vi "ma_SML Decimation Filter (complex input).vi"(2 "reset?":bool, 3 "truncate transition?":bool=TRUE, 4 "decimation setting":T1={"M"=1, "stop band attenuation"=enum."84 dB", "alias protect in transition band"=TRUE, "oversampling ratio"=1.0} {"oversampling ratio" format="%.2f"; "M" min=0}, 5 "x":cdb[](array[numeric]) format="%.2f") -> (0 "initial cutoff length":i32=1 min=0, 1 "y":cdb[](array[numeric]) format="%.2f")   [LabVIEW 2020, in "NI_MAPro.lvlib"]
uses:
  NI_MAPro.lvlib
  NI_AALPro.lvlib
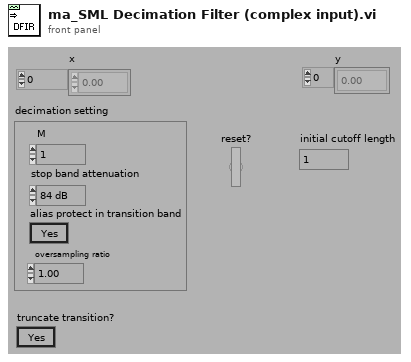
[diagram p1: front panel]
types:
  T1 = cluster{"M":i32, "stop band attenuation":enum16{"84 dB", "96 dB", "120 dB"}, "alias protect in transition band":bool, "oversampling ratio":dbl}
  T2 = cluster{"M":bool, "stop band attenuation":bool, "alias protect in transition band":bool, "oversampling ratio":bool}
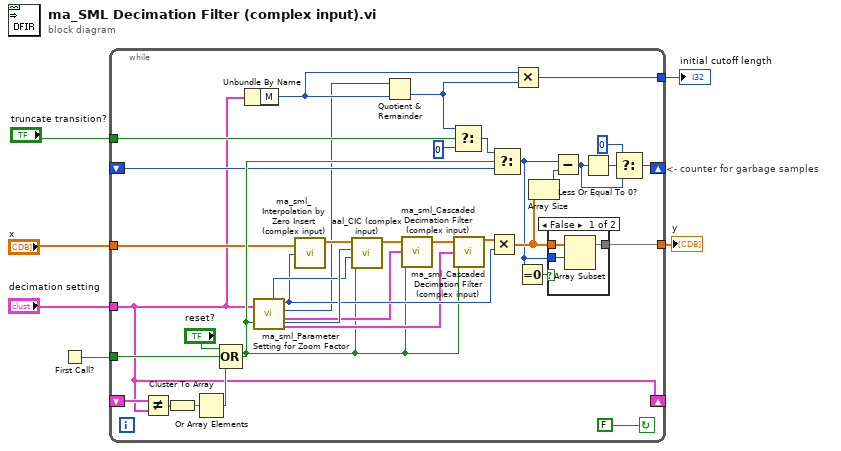
[diagram p0: block diagram]
diagram:
  # "<- counter for garbage samples"
  n1 = First Call?() -> (First Call?: T/F=w3:bool)
  n2 = while {
    tunnel: [w10] -> w1
    tunnel: "truncate transition?" -> [w12]
    tunnel: w3 -> [w13]
    tunnel: "x" -> [w18]
    tunnel: "decimation setting" -> [w11]
    shift-left: _ -> [w27]
    shift-right: [w23] -> _
    tunnel: [w30] -> w6
    shift-left: _ -> [w34]
    shift-right: [w11] -> _
    stop <- FALSE continue-if-true
    n3 = Not Equal?(x=w34, y=w11) -> (x != y?=w33:T2)
    n4 = Cluster To Array(cluster=w33) -> (array=w32:bool[])
    n5 = Or Array Elements(Boolean array=w32) -> (logical OR=w14:bool)
    n6 = Compound Arithmetic op=OR("reset?", w13, w14) -> (w28:bool)
    n7 = Unbundle By Name(w11) -> ("M"=w8:i32)
    n8 = call "ma_sml_Parameter Setting for Zoom Factor.vi"("zoom settings"=w11, "Reset"=w28) -> ("CIC Stages"=w40:i32, "comb filter order"=w41:i32, "interpolation"=w39:i32, "filter length"=w7:i32, "CFIR par"=w29:cluster{"h":dbl[], "M":i32, "N":i32}, "LFIR par"=w35:cluster{"h":dbl[], "M":i32, "N":i32})
    n9 = call "ma_sml_Interpolation by Zero Insert (complex input).vi"("L"=w39, "x"=w18) -> ("y"=w42:cdb[])
    n10 = call "aal_CIC (complex input).vi"("Reset"=w28, "Stages"=w40, "N"=w41, "x"=w42) -> ("y"=w36:cdb[])
    n11 = Quotient & Remainder(x=w7, y=w8) -> (floor(x/y)=w9:i32)  [unwired: 1 out]
    n12 = call "ma_sml_Cascaded Decimation Filter (complex input).vi"("reset?"=w28, "filter specification"=w29, "x"=w36) -> ("y"=w38:cdb[])
    n13 = Select(t=w9, s=w12, f=0) -> (s? t:f=w16:i32)
    n14 = call "ma_sml_Cascaded Decimation Filter (complex input).vi"("reset?"=w28, "filter specification"=w35, "x"=w38) -> ("y"=w37:cdb[])
    n15 = Multiply(x=w37, y=w39) -> (x*y=w26:cdb[])
    n16 = Select(t=w16, s=w28, f=w27) -> (s? t:f=w20:i32)
    n17 = Multiply(x=w8, y=w9) -> (x*y=w10:i32)
    n18 = Equal To 0?(x=w20) -> (x = 0?=w19:bool)
    n19 = Array Size(array=w26) -> (size(s)=w25:i32)
    n20 = case shown="False" w19 {
      tunnel: [w45 w46] -> w30
      tunnel: w26 -> [w44 w46]
      tunnel: w20 -> [w43 _]
      frame False {
        n21 = Array Subset(array=w44, index=w43) -> (w45:cdb[])  [unwired: 1 in]
      }
      frame True {
      }
    }
    n22 = Subtract(x=w20, y=w25) -> (x-y=w22:i32)
    n23 = Less Or Equal To 0?(x=w22) -> (x <= 0?=w24:bool)
    n24 = Select(t=0, s=w24, f=w22) -> (s? t:f=w23:i32)
  }
  "y" <- w6
  "initial cutoff length" <- w1
